vi "dfd_Group Delay_Generate Grid Points.vi"(7 "Order":i32, 9 "grid density":i32=20, 11 "band specification":T1[](array[typedef]) {"subband specs"."weight" format="%.2f"}) -> (0 "weight for grid":dbl[](array[numeric]), 2 "fgrid":dbl[](array[numeric]), 3 "band specification (dup)":T1[](array[typedef]) {"subband specs"."weight" format="%.2f"}, 4 "grid length":dbl)   [LabVIEW 2017, in "NI_DigFilter_Design.lvlib"]
uses:
  <vilib>/addons/Digital Filter Design/NI_DigFilter_Design.lvlib
  <vilib>/addons/Digital Filter Design/_GroupDelay.llb/dfd_Group Delay_Band Spec.ctl
  <vilib>/addons/Digital Filter Design/NI_DigFilterLicensed.lvlib
panel:
  # "freq"
  # "group delay"
  # "weight"
  # "freq"
  # "group delay"
  # "weight"
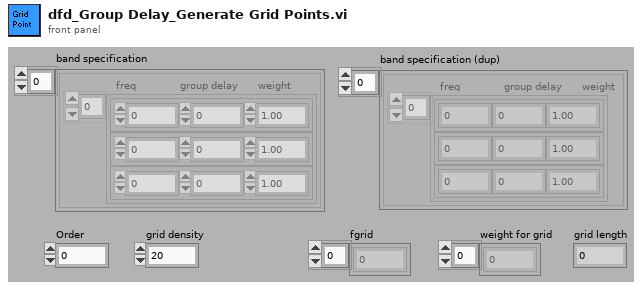
[diagram p1: front panel]
types:
  T1 = typedef "NI_DigFilterLicensed.lvlib/dfd_Group Delay_Band Spec.ctl" = cluster{"subband specs":cluster{"freq":dbl, "group delay":dbl, "weight":dbl}[]}
  T2 = cluster{"freq":dbl, "group delay":dbl, "weight":dbl}[]
  T3 = cluster{"freq":dbl, "group delay":dbl, "weight":dbl}
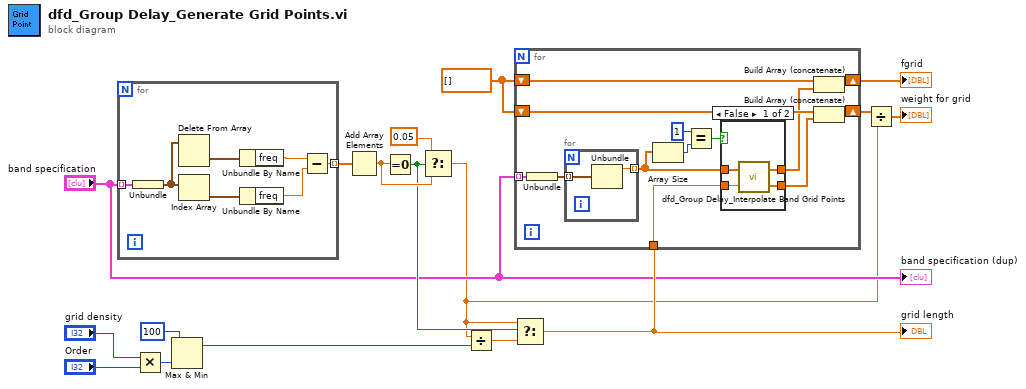
[diagram p0: block diagram]
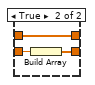
[diagram p2: hidden frame]
diagram:
  w14 = dbl[] []
  n1 = for {
    tunnel: "band specification" -> [w24] mode=indexing
    tunnel: [w21] -> w12 mode=indexing
    n2 = Unbundle(w24) -> ("subband specs"=w20:T2)
    n3 = Delete From Array(array=w20) -> (deleted portion=w23:T3)  [unwired: 2 in, 1 out]
    n4 = Index Array(array=w20) -> (element=w22:T3)  [unwired: 1 in]
    n5 = Unbundle By Name(w23) -> ("freq"=w19:dbl)
    n6 = Unbundle By Name(w22) -> ("freq"=w18:dbl)
    n7 = Subtract(x=w19, y=w18) -> (x-y=w21:dbl)
  }
  n8 = Multiply(x="grid density", y="Order") -> (x*y=w17:i32)
  n9 = Max & Min(x=100, y=w17) -> (max(x,y)=w11:i32)  [unwired: 1 out]
  n10 = Add Array Elements(numeric array=w12) -> (sum=w7:dbl)
  n11 = Equal To 0?(x=w7) -> (x = 0?=w3:bool)
  n12 = Select(t=0.05, s=w3, f=w7) -> (s? t:f=w1:dbl)
  n13 = Divide(x=w1, y=w11) -> (x/y=w4:dbl)
  n14 = Select(t=w1, s=w3, f=w4) -> (s? t:f=w5:dbl)
  "grid length" <- w5
  n15 = for {
    tunnel: "band specification" -> [w37] mode=indexing
    tunnel: w5 -> [w31]
    shift-right: [w34] -> w8
    shift-left: w14 -> [w35]
    shift-right: [w32] -> w13
    shift-left: w14 -> [w33]
    n16 = Unbundle(w37) -> ("subband specs"=w36:T2)
    n17 = for {
      tunnel: w36 -> [w46] mode=indexing
      tunnel: [w45] -> w28 mode=indexing
      n18 = Unbundle(w46) -> ("freq"=w45:dbl)  [unwired: 2 out]
    }
    n19 = Array Size(array=w28) -> (size(s)=w27:i32)
    n20 = Equal?(x=1, y=w27) -> (x = y?=w25:bool)
    n21 = case shown="False" w25 {
      tunnel: w31 -> [w40 w43]
      tunnel: [w39 w44] -> w30
      tunnel: [w38 w42] -> w29
      tunnel: w28 -> [w41 w44]
      frame False {
        n22 = call <vilib>:"dfd_Group Delay_Interpolate Band Grid Points.vi"("nominal df"=w40, "f"=w41) -> ("delta f"=w38:dbl[], "interpolated f"=w39:dbl[])
      }
      frame True {
        n23 = Build Array(w43) -> (w42:dbl[])
      }
    }
    n24 = Build Array (concatenate)(w35, w30) -> (w34:dbl[])
    n25 = Build Array (concatenate)(w33, w29) -> (w32:dbl[])
  }
  "fgrid" <- w8
  n26 = Divide(x=w13, y=w1) -> (x/y=→"weight for grid":dbl[])
  "band specification (dup)" <- "band specification"
